vi "FindGoalDirection.vi"(0 "Start Goal Data in":T1, 5 "Match Index":i32) -> (4 "Start Goal Data out":T1, 6 "x1 4":i32, 8 "x1 3":i32, 10 "x1 2":i32, 15 "x1":i32)   [LabVIEW 2013]
uses:
  Bug_StartGoalData.ctl
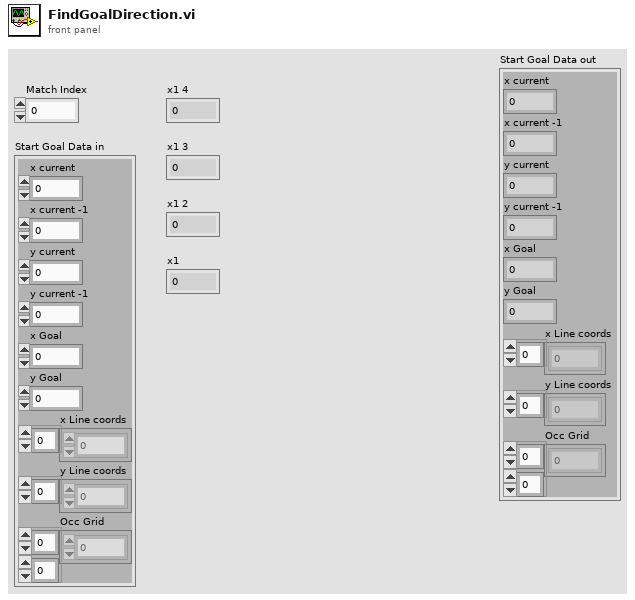
[diagram p1: front panel]
types:
  T1 = typedef "Bug_StartGoalData.ctl" = cluster{"x current":i32, "x current -1":i32, "y current":i32, "y current -1":i32, "x Goal":i32, "y Goal":i32, "x Line coords":i32[], "y Line coords":i32[], "Occ Grid":dbl[][]}
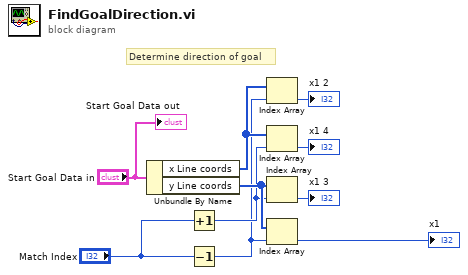
[diagram p0: block diagram]
diagram:
  # "Determine direction of goal"
  n1 = Unbundle By Name("Start Goal Data in") -> ("x Line coords"=w3:i32[], "y Line coords"=w4:i32[])
  n2 = Increment(x="Match Index") -> (x+1=w2:i32)
  n3 = Decrement(x="Match Index") -> (x-1=w1:i32)
  n4 = Index Array(array=w3, index=w1) -> (element=→"x1 2":i32)
  n5 = Index Array(array=w3, index=w2) -> (element=→"x1 4":i32)
  n6 = Index Array(array=w4, index=w2) -> (element=→"x1 3":i32)
  n7 = Index Array(array=w4, index=w1) -> (element=→"x1":i32)
  "Start Goal Data out" <- "Start Goal Data in"
